vi "RowColDecoder.vi"(8 "high  freq":dbl, 11 "low freq":dbl) -> (2 "result":i32)   [LabVIEW 2019]
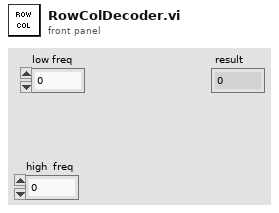
[diagram p1: front panel]
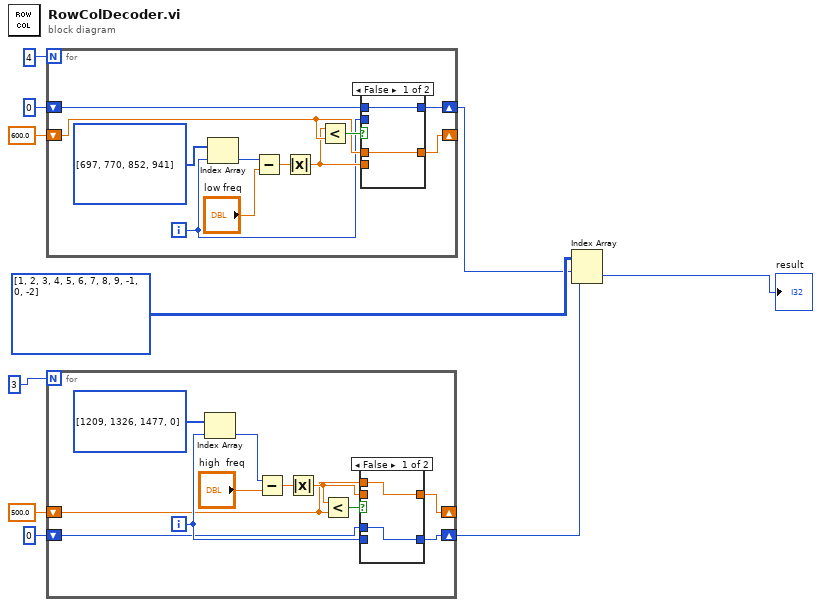
[diagram p0: block diagram]
diagram:
  n1 = for {
    N: 4 -> [_]
    shift-right: [w16] -> _
    shift-left: 600.0 -> [w15]
    shift-right: [w12] -> w3
    shift-left: 0 -> [w11]
    i -> [w13]
    n2 = Index Array(array=i32[] [697, 770, 852, 941], index=w13) -> (element=w20:i32)
    n3 = Subtract(x=w20, y="low freq") -> (x-y=w18:dbl)
    n4 = Absolute Value(x=w18) -> (abs(x)=w14:dbl)
    n5 = Less?(x=w14, y=w15) -> (x < y?=w17:bool)
    n6 = case shown="False" w17 {
      tunnel: [w23 w25] -> w16
      tunnel: w15 -> [w23 _]
      tunnel: w14 -> [_ w25]
      tunnel: w13 -> [_ w24]
      tunnel: [w22 w24] -> w12
      tunnel: w11 -> [w22 _]
      frame False {
      }
      frame True {
      }
    }
  }
  n7 = for {
    N: 3 -> [_]
    shift-right: [w30] -> _
    shift-left: 500.0 -> [w26]
    shift-right: [w28] -> w2
    shift-left: 0 -> [w27]
    i -> [w29]
    n8 = Index Array(array=i32[] [1209, 1326, 1477, 0], index=w29) -> (element=w35:i32)
    n9 = Subtract(x=w35, y="high  freq") -> (x-y=w33:dbl)
    n10 = Absolute Value(x=w33) -> (abs(x)=w31:dbl)
    n11 = Less?(x=w31, y=w26) -> (x < y?=w32:bool)
    n12 = case shown="False" w32 {
      tunnel: w31 -> [_ w40]
      tunnel: [w37 w40] -> w30
      tunnel: w29 -> [_ w39]
      tunnel: [w38 w39] -> w28
      tunnel: w27 -> [w38 _]
      tunnel: w26 -> [w37 _]
      frame False {
      }
      frame True {
      }
    }
  }
  n13 = Index Array(array=i32[][] [[1, 2, 3], [4, 5, 6], [7, 8, 9], [-1, 0, -2]], index (row)=w3, index (col)=w2) -> (element=→"result":i32)
